vi "Op-Graphics-Cursor.vi"(5 "Y axis":bool, 6 "Y position":dbl format="%^.4e", 7 "X position":dbl format="%^.4e", 8 "error in (no error)":errorcluster, 9 "cursor state (off:0)":u8(ring) items=["off", "short", "long"], 10 "move cursor to":bool, 11 "VISA session":refnum<visa-resource-name>) -> (0 "error out":errorcluster, 3 "VISA resource name out":refnum<visa-resource-name>)   [LabVIEW 2016, in "Agilent 415X Series.lvlib"]
doc: "This VI sets the state of the graphical cursor used with the GRAPHICS display mode. Also this VI moves the cursor to the desired location."
uses:
  Agilent 415X Series.lvlib
panel:
  # "This VI will change the display mode to GRAPHICS"
  # "on"
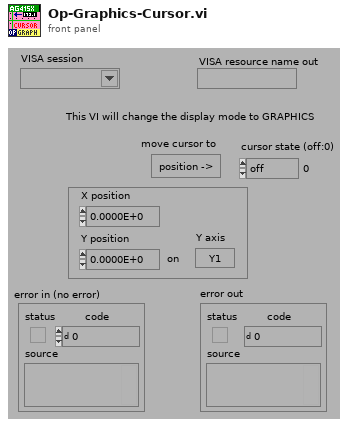
[diagram p1: front panel]
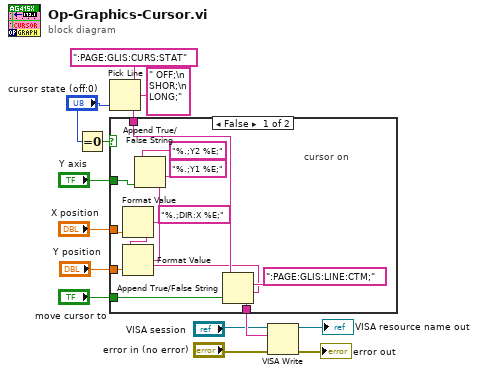
[diagram p0: block diagram]
diagram:
  n1 = Equal To 0?(x="cursor state (off:0)") -> (x = 0?=w13:bool)
  n2 = Pick Line(string ("")=":PAGE:GLIS:CURS:STAT", multi-line string=" OFF;\n SHOR;\n LONG;", line index="cursor state (off:0)") -> (output string=w8:string)
  n3 = case shown="False" w13 {
    tunnel: "Y axis" -> [w20 _]
    tunnel: "X position" -> [w27 _]
    tunnel: w8 -> [w25 w28]
    tunnel: "move cursor to" -> [w22 _]
    tunnel: [w23 w28] -> w6
    tunnel: "Y position" -> [w21 _]
    frame False {
      # "cursor on"
      n4 = Format Value(format string="%.;DIR:X %E;", value (0)=w27) -> (output string=w16:string)  [unwired: 1 in]
      n5 = Append True/False String(1:w20, 2:"%.;Y1 %E;", 3:"%.;Y2 %E;") -> (0:w17:string)  [unwired: 1 in]
      n6 = Format Value(string ("")=w16, format string=w17, value (0)=w21) -> (output string=w15:string)
      n7 = Append True/False String(1:w22, 2:w15, 3:":PAGE:GLIS:LINE:CTM;", 4:w25) -> (0:w23:string)
    }
    frame True {
      # "cursor off"
    }
  }
  n8 = VISA Write(VISA resource name="VISA session", write buffer=w6, error in (no error)="error in (no error)") -> (VISA resource name out=→"VISA resource name out":refnum<visa-resource-name>, error out=→"error out":errorcluster)  [unwired: 1 out]
